vi "Data Logging_Generate Header.vi"(8 "error in":errorcluster, 9 "Include Units\nin Header (F)":bool, 10 "Units of Measure Input":T2, 11 "Data Logging Options":T1={"Absolute Press."=TRUE, "Gauge/Diff. Press."=TRUE, "Barometric Press."=TRUE, "Temperature"=TRUE, "Volumetric"=TRUE, "Mass Flow"=TRUE, "Setpoint"=FALSE, "Valve Drive"=FALSE, "Totalizer"=TRUE, "Tot. Timer [s]"=TRUE, "Tot. Avg. Flow"=TRUE, "Tot. Peak Flow"=TRUE, "Gas Selected"=TRUE, "Log Data"=FALSE}) -> (0 "error out":errorcluster, 2 "Header Array":string[](array[string]), 3 "Data Log Header":string)   [LabVIEW 2016]
doc: "Generates a header string for use with data logging. Output will be a comma delimited string containing labels of the variables (and the units of measure, if selected) for the data logging options selected."
uses:
  Units of Measure.ctl
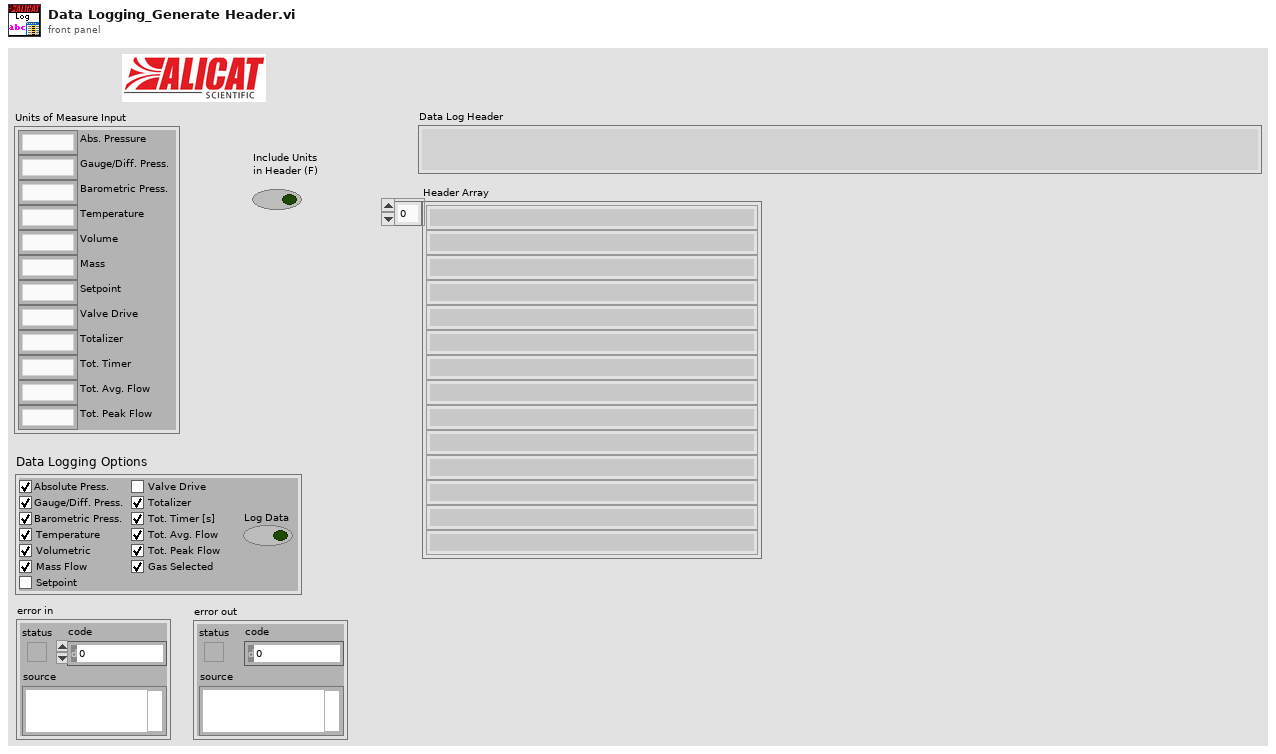
[diagram p1: front panel]
types:
  T1 = cluster{"Absolute Press.":bool, "Gauge/Diff. Press.":bool, "Barometric Press.":bool, "Temperature":bool, "Volumetric":bool, "Mass Flow":bool, "Setpoint":bool, "Valve Drive":bool, "Totalizer":bool, "Tot. Timer [s]":bool, "Tot. Avg. Flow":bool, "Tot. Peak Flow":bool, "Gas Selected":bool, "Log Data":bool}
  T2 = typedef "Units of Measure.ctl" = cluster{"Abs. Pressure":string, "Gauge/Diff. Press.":string, "Barometric Press.":string, "Temperature":string, "Volume":string, "Mass":string, "Setpoint":string, "Valve Drive":string, "Totalizer":string, "Tot. Timer":string, "Tot. Avg. Flow":string, "Tot. Peak Flow":string}
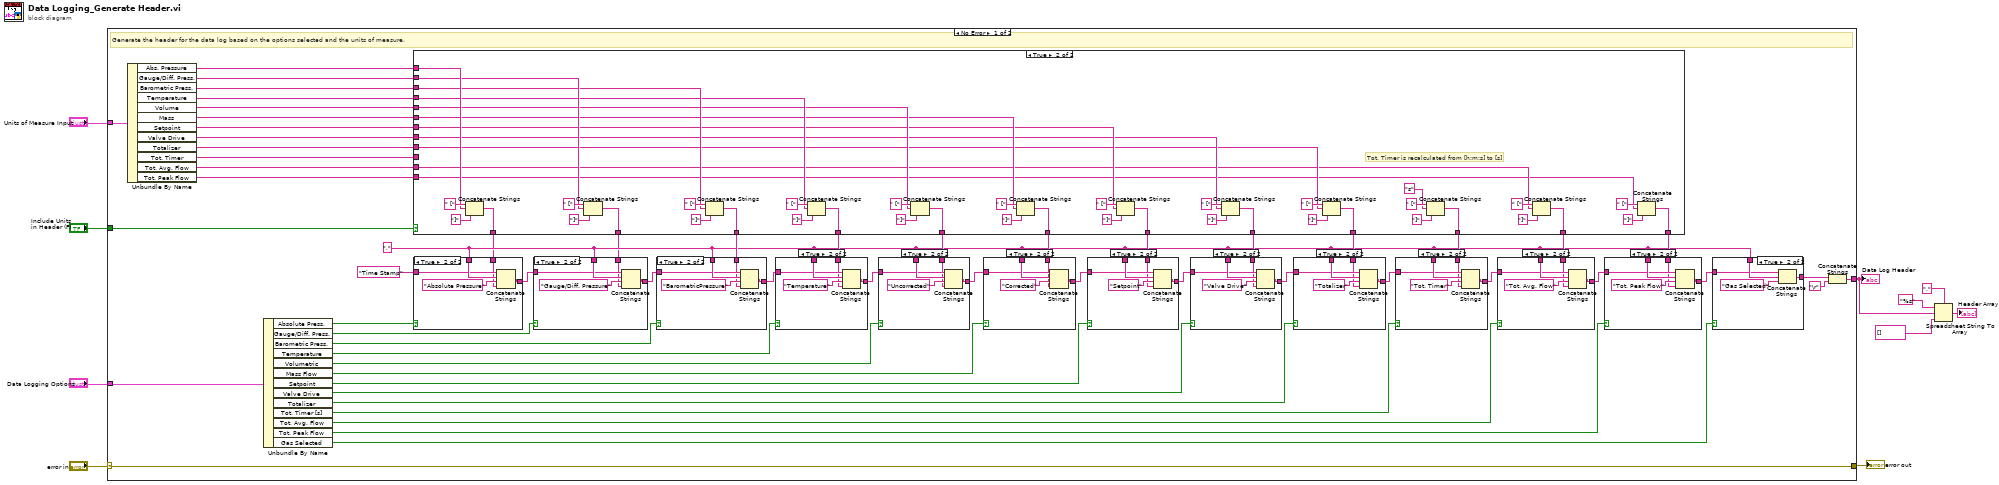
[diagram p0: block diagram]
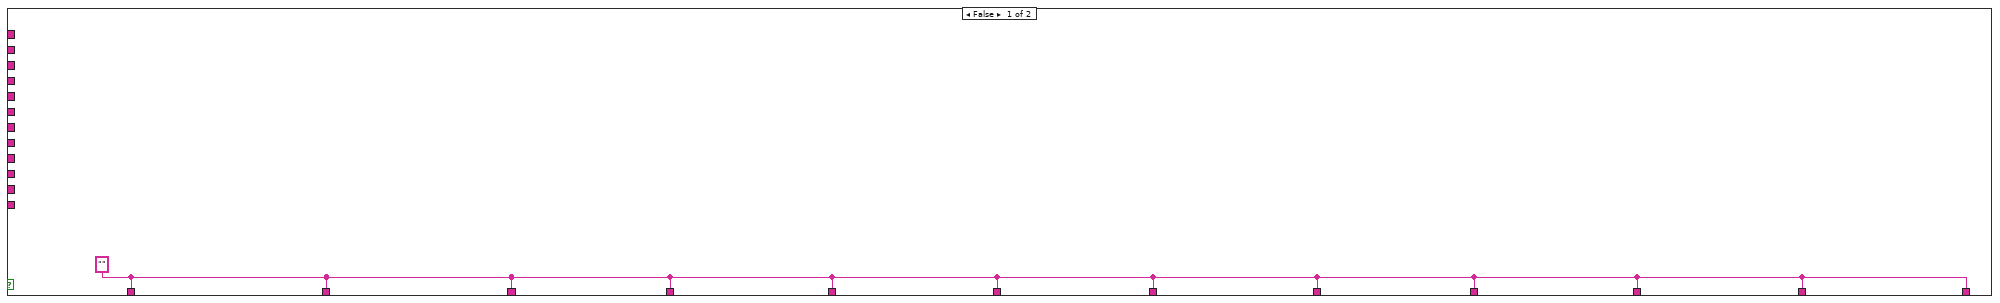
[diagram p4: hidden frame]
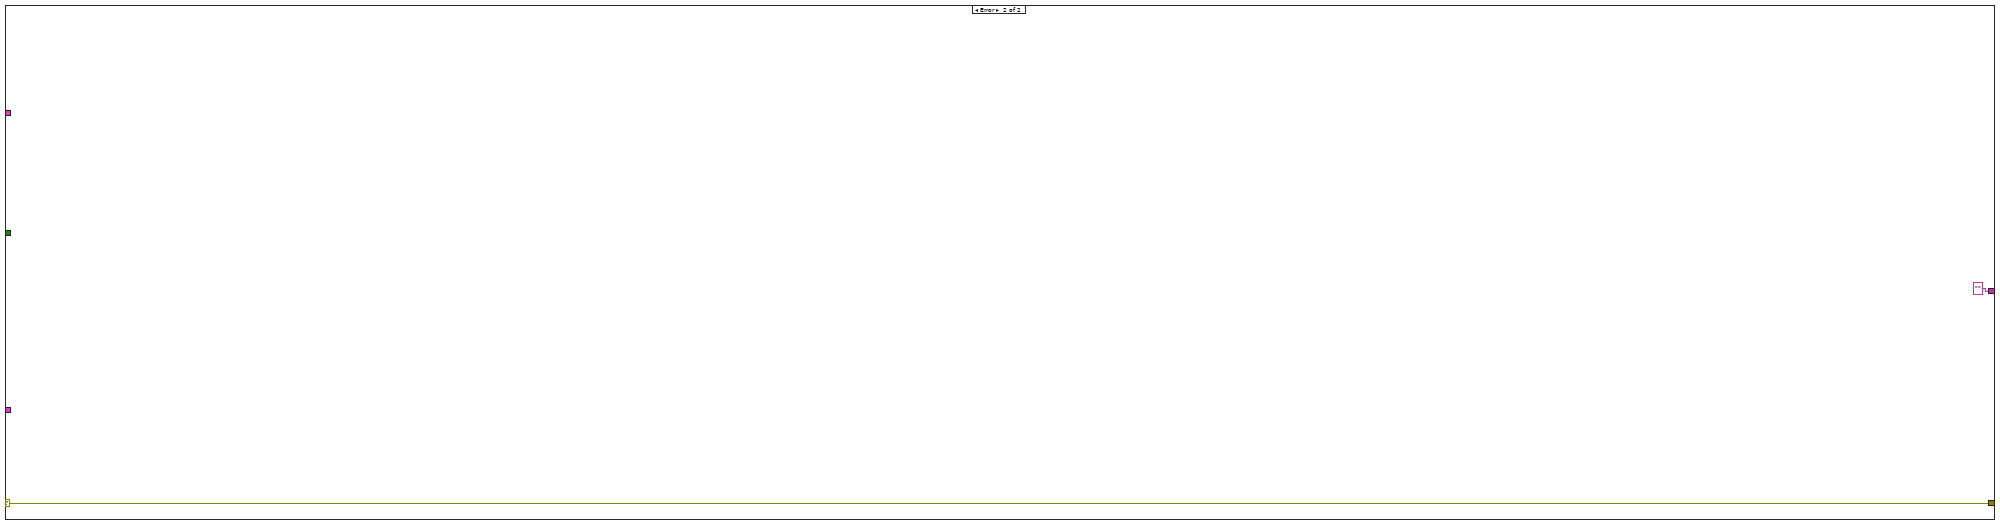
[diagram p16: hidden frame]
diagram:
  n1 = case shown="No Error" "error in" {
    selector: "error in" -> [w47 w195]
    tunnel: "Data Logging Options" -> [w48 _]
    tunnel: [w47 w195] -> w9
    tunnel: "Units of Measure Input" -> [w32 _]
    tunnel: [w45 "" ("string")] -> w5
    tunnel: "Include Units\nin Header (F)" -> [w33 _]
    frame No Error {
      w29 = "," ("string")
      # "Generate the header for the data log based on the options selected and the units of measure."
      n2 = Unbundle By Name(w32) -> ("Abs. Pressure"=w13:string, "Gauge/Diff. Press."=w14:string, "Barometric Press."=w15:string, "Temperature"=w16:string, "Volume"=w17:string, "Mass"=w18:string, "Setpoint"=w19:string, "Valve Drive"=w20:string, "Totalizer"=w21:string, "Tot. Timer"=w22:string, "Tot. Avg. Flow"=w23:string, "Tot. Peak Flow"=w24:string)
      n3 = Unbundle By Name(w48) -> ("Absolute Press."=w27:bool, "Gauge/Diff. Press."=w25:bool, "Barometric Press."=w26:bool, "Temperature"=w58:bool, "Volumetric"=w57:bool, "Mass Flow"=w56:bool, "Setpoint"=w55:bool, "Valve Drive"=w54:bool, "Totalizer"=w53:bool, "Tot. Timer [s]"=w52:bool, "Tot. Avg. Flow"=w51:bool, "Tot. Peak Flow"=w50:bool, "Gas Selected"=w49:bool)
      n4 = case shown="True" w33 {
        tunnel: [w81 w129] -> w43
        tunnel: [w81 w124] -> w42
        tunnel: [w81 w123] -> w41
        tunnel: [w81 w118] -> w39
        tunnel: [w81 w100] -> w40
        tunnel: [w81 w113] -> w38
        tunnel: [w81 w112] -> w37
        tunnel: [w81 w107] -> w36
        tunnel: [w81 w106] -> w35
        tunnel: [w81 w101] -> w34
        tunnel: w24 -> [_ w85]
        tunnel: w23 -> [_ w86]
        tunnel: w22 -> [_ _]
        tunnel: w21 -> [_ w87]
        tunnel: w20 -> [_ w88]
        tunnel: w19 -> [_ w89]
        tunnel: w18 -> [_ w90]
        tunnel: w17 -> [_ w91]
        tunnel: w16 -> [_ w92]
        tunnel: w15 -> [_ w93]
        tunnel: w14 -> [_ w94]
        tunnel: w13 -> [_ w95]
        tunnel: [w81 w83] -> w12
        tunnel: [w81 w82] -> w11
        frame False {
          w81 = ""
          # "no units of measure included"
        }
        frame True {
          # "Tot. Timer is recalculated from [h:m:s] to [s]"
          # "Get the units of measure, if enabled"
          n5 = Concatenate Strings(" [" ("string"), w95, "]" ("string")) -> (w82:string)
          n6 = Concatenate Strings(" [" ("string"), w94, "]" ("string")) -> (w83:string)
          n7 = Concatenate Strings(" [" ("string"), w93, "]" ("string")) -> (w129:string)
          n8 = Concatenate Strings(" [" ("string"), w92, "]" ("string")) -> (w124:string)
          n9 = Concatenate Strings(" [" ("string"), w91, "]" ("string")) -> (w123:string)
          n10 = Concatenate Strings(" [" ("string"), w90, "]" ("string")) -> (w118:string)
          n11 = Concatenate Strings(" [" ("string"), w89, "]" ("string")) -> (w100:string)
          n12 = Concatenate Strings(" [" ("string"), w88, "]" ("string")) -> (w113:string)
          n13 = Concatenate Strings(" [" ("string"), w87, "]" ("string")) -> (w112:string)
          n14 = Concatenate Strings(" [" ("string"), "s" ("string"), "]" ("string")) -> (w107:string)
          n15 = Concatenate Strings(" [" ("string"), w86, "]" ("string")) -> (w106:string)
          n16 = Concatenate Strings(" [" ("string"), w85, "]" ("string")) -> (w101:string)
        }
      }
      n17 = case shown="True" w27 {
        tunnel: "Time Stamp" ("string") -> [w69 w71]
        tunnel: [w69 w74] -> w31
        tunnel: w29 -> [_ w72]
        tunnel: w11 -> [_ w70]
        frame False {
        }
        frame True {
          n18 = Concatenate Strings(w71, w72, "Absolute Pressure" ("string"), w70) -> (w74:string)
        }
      }
      n19 = case shown="True" w25 {
        tunnel: w31 -> [w75 w77]
        tunnel: [w75 w80] -> w30
        tunnel: w29 -> [_ w78]
        tunnel: w12 -> [_ w76]
        frame False {
        }
        frame True {
          n20 = Concatenate Strings(w77, w78, "Gauge/Diff. Pressure" ("string"), w76) -> (w80:string)
        }
      }
      n21 = case shown="True" w26 {
        tunnel: w30 -> [w189 w191]
        tunnel: [w189 w194] -> w68
        tunnel: w29 -> [_ w192]
        tunnel: w43 -> [_ w190]
        frame False {
        }
        frame True {
          n22 = Concatenate Strings(w191, w192, "BarometricPressure" ("string"), w190) -> (w194:string)
        }
      }
      n23 = case shown="True" w58 {
        tunnel: w68 -> [w183 w185]
        tunnel: [w183 w188] -> w60
        tunnel: w29 -> [_ w186]
        tunnel: w42 -> [_ w184]
        frame False {
        }
        frame True {
          n24 = Concatenate Strings(w185, w186, "Temperature" ("string"), w184) -> (w188:string)
        }
      }
      n25 = case shown="True" w57 {
        tunnel: w60 -> [w177 w179]
        tunnel: [w177 w182] -> w59
        tunnel: w29 -> [_ w180]
        tunnel: w41 -> [_ w178]
        frame False {
        }
        frame True {
          n26 = Concatenate Strings(w179, w180, "Uncorrected" ("string"), w178) -> (w182:string)
        }
      }
      n27 = case shown="True" w56 {
        tunnel: w59 -> [w171 w173]
        tunnel: [w171 w176] -> w67
        tunnel: w29 -> [_ w174]
        tunnel: w39 -> [_ w172]
        frame False {
        }
        frame True {
          n28 = Concatenate Strings(w173, w174, "Corrected" ("string"), w172) -> (w176:string)
        }
      }
      n29 = case shown="True" w55 {
        tunnel: w67 -> [w165 w167]
        tunnel: [w165 w170] -> w66
        tunnel: w29 -> [_ w168]
        tunnel: w40 -> [_ w166]
        frame False {
        }
        frame True {
          n30 = Concatenate Strings(w167, w168, "Setpoint" ("string"), w166) -> (w170:string)
        }
      }
      n31 = case shown="True" w54 {
        tunnel: w66 -> [w159 w161]
        tunnel: [w159 w164] -> w65
        tunnel: w29 -> [_ w162]
        tunnel: w38 -> [_ w160]
        frame False {
        }
        frame True {
          n32 = Concatenate Strings(w161, w162, "Valve Drive" ("string"), w160) -> (w164:string)
        }
      }
      n33 = case shown="True" w53 {
        tunnel: w65 -> [w153 w155]
        tunnel: [w153 w158] -> w64
        tunnel: w29 -> [_ w156]
        tunnel: w37 -> [_ w154]
        frame False {
        }
        frame True {
          n34 = Concatenate Strings(w155, w156, "Totalizer" ("string"), w154) -> (w158:string)
        }
      }
      n35 = case shown="True" w52 {
        tunnel: w64 -> [w147 w149]
        tunnel: [w147 w152] -> w63
        tunnel: w29 -> [_ w150]
        tunnel: w36 -> [_ w148]
        frame False {
        }
        frame True {
          n36 = Concatenate Strings(w149, w150, "Tot. Timer" ("string"), w148) -> (w152:string)
        }
      }
      n37 = case shown="True" w51 {
        tunnel: w63 -> [w141 w143]
        tunnel: [w141 w146] -> w62
        tunnel: w29 -> [_ w144]
        tunnel: w35 -> [_ w142]
        frame False {
        }
        frame True {
          n38 = Concatenate Strings(w143, w144, "Tot. Avg. Flow" ("string"), w142) -> (w146:string)
        }
      }
      n39 = case shown="True" w50 {
        tunnel: w62 -> [w135 w137]
        tunnel: [w135 w140] -> w61
        tunnel: w29 -> [_ w138]
        tunnel: w34 -> [_ w136]
        frame False {
        }
        frame True {
          n40 = Concatenate Strings(w137, w138, "Tot. Peak Flow" ("string"), w136) -> (w140:string)
        }
      }
      n41 = case shown="True" w49 {
        tunnel: w61 -> [w130 w131]
        tunnel: [w130 w134] -> w46
        tunnel: w29 -> [_ w132]
        frame False {
        }
        frame True {
          n42 = Concatenate Strings(w131, w132, "Gas Selected" ("string")) -> (w134:string)
        }
      }
      n43 = Concatenate Strings(w46, "\r" ("string")) -> (w45:string)
    }
    frame Error {
    }
  }
  "error out" <- w9
  "Data Log Header" <- w5
  n44 = Spreadsheet String To Array(delimiter (Tab)=",", format string="%s", spreadsheet string=w5, array type (2D Dbl)=string[] []) -> (array=→"Header Array":string[])
